vi "Inverse Time Curves (IEEE, Definite Reset).vi"(6 "operate time compensation":cluster{"G/Gs":dbl, "compensation [s]":dbl}[](array[cluster]), 7 "GD (25)":u16=25, 8 "error in (no error)":errorcluster, 9 "reset delay (0 s)":dbl, 10 "time multiplier setting (1)":dbl=1.0, 11 "curve type":u16(ring) items=["IEEE moderately inverse", "IEEE very inverse", "IEEE extremely inverse"]) -> (0 "error out":errorcluster, 2 "memory size":u16, 3 "memory initial values":fxp<+,51,51>[](array[numeric]), 4 "curve data":cluster{"G/Gs":dbl[], "times [s]":dbl[]})   [LabVIEW 2014, in "NI_EP_Protection.lvlib"]
doc: "Generates memory initial values and memory size, which contain the information of the inverse time curves, for the FPGA Inverse Time Delay VI to use. You can compensate for the processing delay of the input energizing quantity under a specific G/Gs to achieve higher operate time accuracy."
uses:
  <vilib>/addons/Electrical Power/Protection/NI_EP_Protection.lvlib
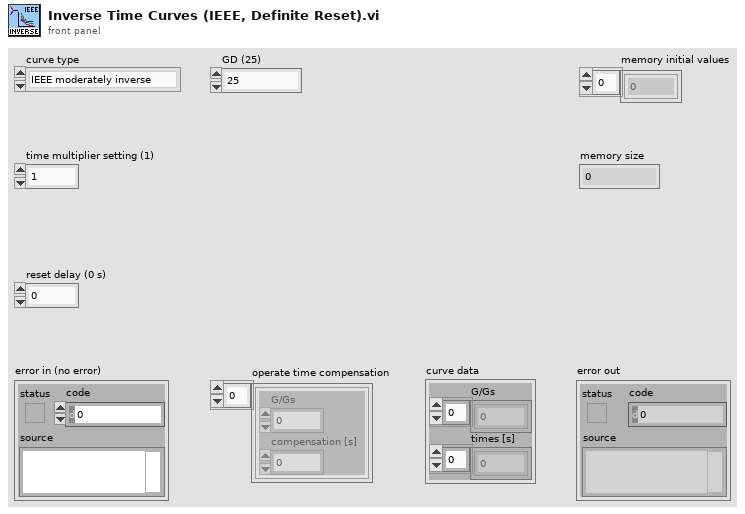
[diagram p1: front panel]
types:
  T1 = typedef "NI_EP_Protection.lvlib/ep_Curve Parameters.ctl" = cluster{"operate time parameters":T2, "reset time parameters":T3}
  T2 = typedef "NI_EP_Protection.lvlib/ep_Operate Time.ctl" = cluster{"A [s]":dbl, "B [s]":dbl, "alpha":dbl, "K2 [s]":dbl, "K1 [s]":dbl, "K3 [s]":dbl}
  T3 = typedef "NI_EP_Protection.lvlib/ep_Reset Time.ctl" = cluster{"tr [s]":dbl, "alpha":dbl}
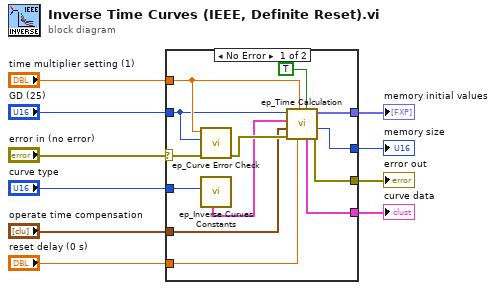
[diagram p0: block diagram]
diagram:
  n1 = case shown="No Error" "error in (no error)" {
    selector: "error in (no error)" -> [w21 w24]
    tunnel: [w16 w24] -> w9
    tunnel: "curve type" -> [w18 _]
    tunnel: "GD (25)" -> [w22 _]
    tunnel: "time multiplier setting (1)" -> [w23 _]
    tunnel: [w19 _] -> w5
    tunnel: [w17 _] -> w4
    tunnel: [w15 _] -> w3
    tunnel: "reset delay (0 s)" -> [w14 _]
    tunnel: "operate time compensation" -> [w11 _]
    frame No Error {
      n2 = call <vilib>:"ep_Curve Error Check.vi"("error in (no error)"=w21, "GD"=w22, "time dial"=w23) -> ("error out"=w20:errorcluster)  [unwired: 8 in]
      n3 = call <vilib>:"ep_Inverse Curves Constants.vi"("IEEE curve type"=w18) -> ("IEEE parameters"=w12:T1)  [unwired: 5 in, 5 out]
      n4 = call <vilib>:"ep_Time Calculation.vi"("definite reset? (F)"=TRUE, "reset delay [s]"=w14, "time dial"=w23, "error in (no error)"=w20, "operate time compensation"=w11, "curve parameters"=w12, "GD"=w22) -> ("error out"=w16:errorcluster, "memory size"=w19:u16, "memory initial values"=w17:fxp<+,51,51>[], "curve data"=w15:cluster{"G/Gs":dbl[], "times":dbl[]})  [unwired: 1 in]
    }
    frame Error {
    }
  }
  "memory initial values" <- w4
  "error out" <- w9
  "memory size" <- w5
  "curve data" <- w3
